vi "CRYData View Legend New Insert.vi"(6 "Item Symbols":i32[](array[numeric]), 8 "Color Array":u32[](array[colorbox]), 9 "ItemName Array":string[](array[string]), 10 "sOption":string, 11 "pGraph VI In":refnum<vi>) -> (3 "pGraph VI Out":refnum<vi>)   [LabVIEW 2013]
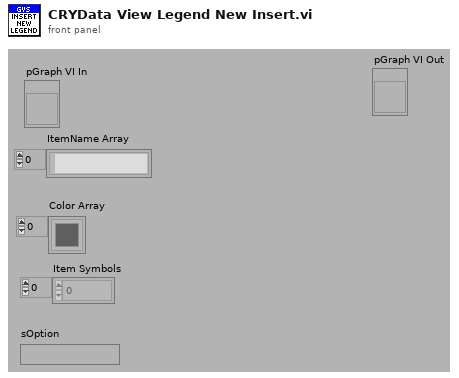
[diagram p1: front panel]
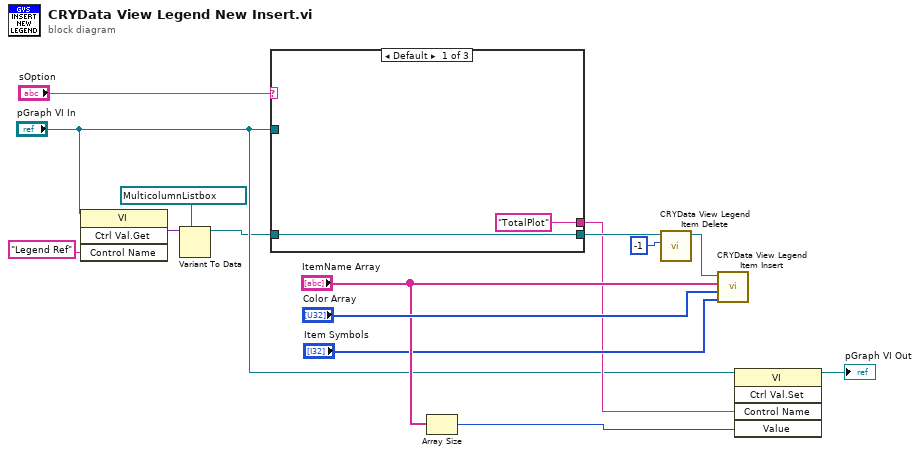
[diagram p0: block diagram]
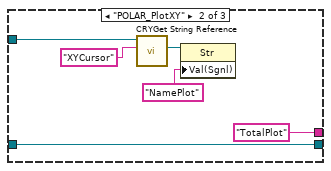
[diagram p2: hidden frame]
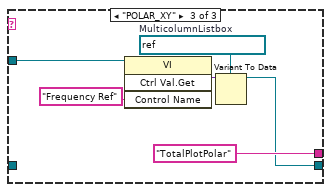
[diagram p3: hidden frame]
diagram:
  n1 = invoke class="VI" method="Ctrl Val.Get"(reference="pGraph VI In", "Control Name"="Legend Ref") -> ("Get Control Value Variant"=w4:variant)  [unwired: 2 in, 3 out]
  n2 = Variant To Data(type=refnum<vi> refnum ("GMListbox"), Variant=w4) -> (data=w1:refnum<vi>)  [unwired: 1 in, 1 out]
  n3 = case shown="Default" "sOption" {
    tunnel: "pGraph VI In" -> [_ w18 w25]
    tunnel: w1 -> [w17 w23 _]
    tunnel: [w17 w23 w24] -> w8
    tunnel: ["TotalPlot" ("Control Name") "TotalPlot" ("Control Name") "TotalPlotPolar" ("Control Name")] -> w7
    frame Default {
    }
    frame "POLAR_PlotXY" {
      n4 = call "CRYGet String Reference.vi"("Label Name"="XYCursor", "VI Refnum"=w18) -> ("String Ref Out"=w21:refnum<vi>)  [unwired: 7 in, 2 out]
      n5 = property class="Str"(reference=w21, "Val(Sgnl)"="NamePlot" ("Value (Signaling)")) -> ()  [unwired: 1 in, 2 out]
    }
    frame "POLAR_XY" {
      w26 = refnum<vi> refnum  # MulticolumnListbox
      n6 = invoke class="VI" method="Ctrl Val.Get"(reference=w25, "Control Name"="Frequency Ref") -> ("Get Control Value Variant"=w28:variant)  [unwired: 2 in, 3 out]
      n7 = Variant To Data(type=w26, Variant=w28) -> (data=w24:refnum<vi>)  [unwired: 1 in, 1 out]
    }
  }
  n8 = Array Size(array="ItemName Array") -> (size(s)=w11:i32)
  n9 = call "CRYData View Legend Item Delete.vi"("RowNumber"=-1, "Legend MultiListbox In"=w8) -> ("Legend MultiListbox Out"=w14:refnum<vi>)  [unwired: 9 out]
  n10 = call "CRYData View Legend Item Insert.vi"("Item Symbols"="Item Symbols", "Color Array"="Color Array", "ItemName Array"="ItemName Array", "Legend MultiListbox"=w14) -> ()  [unwired: 8 out]
  n11 = invoke class="VI" method="Ctrl Val.Set"(reference="pGraph VI In", "Control Name"=w7, "Value"=w11) -> (reference out=→"pGraph VI Out":refnum<vi>)  [unwired: 2 in, 4 out]
